vi "Configure Frequency Shift.vi"(0 "niUsrpRio session":T1 {"Daughterboard Clock Rate" format="%#.3pHz"; "FPGA Data Clock Rate" format="%#.3pHz"; "Data Clock Rate" format="%#.3pHz"; "Characterization Data"."Frequencies [Hz]" format="%#_6p"; "EEPROM Characterization Header"."Pointer to Device Data Header" format="%x"; "EEPROM Characterization Header"."Checksum" format="%x"; "Device Data Header"."Pointer to Characterization Data" format="%x"; "Device Data Header"."Checksum" format="%x"; "EEPROM Header"."Pointer to User Header" format="%x"; "EEPROM Header"."Pointer to Factory Header" format="%x"; "EEPROM Header"."Product Code" format="%x"; "EEPROM Header"."Checksum" format="%x"}, 1 "scope":string(combo)="rx", 5 "clock rate":dbl=120000000.0 format="%#.3pHz", 7 "frequency shift":dbl format="%#.3pHz", 11 "error in":errorcluster) -> (4 "niUsrpRio Session (out)":T1={"FPGA Interface"=refnum, "RIO Interface Number"=0, "Data Clock Rate"=0, "FPGA Data Clock Rate"=0, "Global Settings Register Bus"=refnum, "Radio 0 Settings Register Bus"=refnum, "Radio 1 Settings Register Bus"=refnum, "Radio Settings Bus Semaphore"=refnum, "DB Queues"=[], "Characterization Data Valid?"=FALSE, "EEPROM Header"={"Checksum"=0, "Product Code"=0, "Hardware Current Version"=0, "Hardware Oldest Compatible Version"=0, "EEPROM Map Current Version"=0, "EEPROM Map Oldest Compatible Version"=0, "User Password"="", "Pointer to Factory Header"=0, "Pointer to User Header"=0, "Recommended Interval"=0, "Number of Reserved Bytes"=9, "Number of Daughterboards"=0, "Daughterboard IDs"=[], "Daughterboard Serial Numbers"=[]}, "Device Data Header"={"Checksum"=0, "Number of Channels"=0, "Number of Gain Settings"=[], "Pointer to Characterization Data"=[], "Number of Reserved Bytes"=27, "Number of Frequencies"=[]}, "EEPROM Characterization Header"={"Checksum"=0, "Date"=timestamp(0 s since 1904-01-01), "Temperature"=0.0, "Misc. Info"="", "Pointer to Device Data Header"=0, "Number of Reserved Bytes"=28}, "Characterization Data"=[], "FPGA Current Version"=0, "FPGA Oldest Compatible Version"=0, "Fixed Logic Current Version"=0, "Fixed Logic Oldest Compatible Version"=0, "FPGA Radio Settings Bus Current Version"=0, "FPGA Radio Settings Bus Oldest Compatible Version"=0, "FPGA Board Config Current Version"=0, "FPGA Board Config Oldest Compatible Version"=0, "Daughterboard Clock Rate"=0} {"Daughterboard Clock Rate" format="%#.3pHz"; "FPGA Data Clock Rate" format="%#.3pHz"; "Data Clock Rate" format="%#.3pHz"; "Characterization Data"."Frequencies [Hz]" format="%#_6p"; "EEPROM Characterization Header"."Pointer to Device Data Header" format="%x"; "EEPROM Characterization Header"."Checksum" format="%x"; "Device Data Header"."Pointer to Characterization Data" format="%x"; "Device Data Header"."Checksum" format="%x"; "EEPROM Header"."Pointer to User Header" format="%x"; "EEPROM Header"."Pointer to Factory Header" format="%x"; "EEPROM Header"."Product Code" format="%x"; "EEPROM Header"."Checksum" format="%x"}, 8 "coerced frequency shift":dbl format="%#.3pHz", 15 "error out":errorcluster)   [LabVIEW 2015]
doc: "Configures the digital frequency shift amount.\n\n<B>Input Parameters</B>\n\n<B>niUsrpRio Session</B> is the object created by the Open VI and used as the session handle for the USRP RIO design library.\n\n<B>clock rate</B> is the frequency, in hertz, at which the DSP blocks run.\n\n<B>frequency shift</B> is the amount, in hertz, by which to shift the frequency.\n\n<B>error in</B> describes error conditions that occur before this node runs. This input provides standard 'error in' functionality.\n\n<B>Output Parameters</B>\n\n<B>error out</B> contains error information. This output provides standard 'error out' functionality."
uses:
  <instrlib>/niUsrpRio/Config/v1/Host/Public/niUsrpRio Session.ctl
  <instrlib>/_niInstr/Register Bus/v0/Host/Public/Register Bus Session.ctl
  <instrlib>/_niInstr/Register Bus/v0/Host/Private/Session Data.ctl
  <instrlib>/niUsrpRio/Config/v1/Host/Private/DB Queue Reference.ctl
  <instrlib>/niUsrpRio/Config/v1/Host/Private/Daughterboard Data.ctl
  <instrlib>/niUsrpRio/Config/v1/Host/Private/ATR state data.ctl
  <instrlib>/niUsrpRio/Config/v1/Host/Private/Antenna Configuration.ctl
  <instrlib>/niUsrpRio/Config/v1/Host/Private/CPLD Power Mode.ctl
  <instrlib>/niUsrpRio/Config/v1/Host/Public/EEPROM Header.ctl
  <instrlib>/niUsrpRio/Config/v1/Host/Public/EEPROM Device Data Header.ctl
  <instrlib>/niUsrpRio/Config/v1/Host/Public/EEPROM Characterization Header.ctl
  <instrlib>/niUsrpRio/Config/v1/Host/Public/Characterization Data.ctl
  <instrlib>/niUsrpRio/Config/v1/Host/Public/IQ Imbalance.ctl
  Streaming Xvcr FPGA Ref.ctl
  FPGA/SubVIs/DDC Parameters.ctl
  <instrlib>/_niInstr/DSP/v1/Shared/Public/IQ Impairments.ctl
  <vilib>/rvi/errors/niLvFpgaAdjustHostInterfaceError.vi
  <vilib>/Utility/error.llb/Error Cluster From Error Code.vi
  <vilib>/rvi/interface/nirviReadWriteControl/nirviReadWriteControl.xnode
  NiFpgaLv.dll
  <vilib>/rvi/interface/Simulation/niFpgaSimulationCallBeginRW.vi
  <instrlib>/niUsrpRio/Config/v1/Host/niUsrpRio Config v1 Host.lvlib
  <instrlib>/_niInstr/DSP/v1/Shared/niInstr DSP v1 Shared.lvlib
  <instrlib>/_niInstr/Register Bus/v0/Host/niInstr Register Bus v0 Host.lvlib
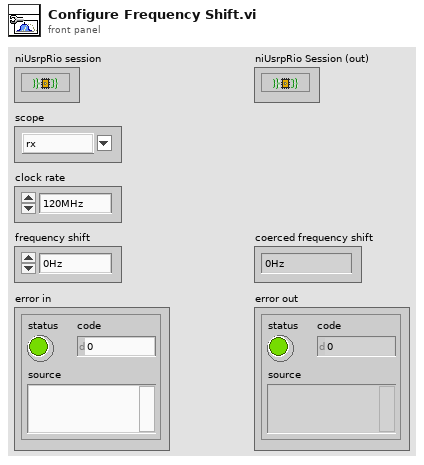
[diagram p1: front panel]
types:
  T1 = typedef "niUsrpRio Config v1 Host.lvlib/niUsrpRio Session.ctl" = cluster{"FPGA Interface":refnum<k20>, "RIO Interface Number":u32, "Data Clock Rate":u32, "FPGA Data Clock Rate":u32, "Global Settings Register Bus":T2, "Radio 0 Settings Register Bus":T2, "Radio 1 Settings Register Bus":T2, "Radio Settings Bus Semaphore":T3, "DB Queues":T4[], "Characterization Data Valid?":bool, "EEPROM Header":T5, "Device Data Header":T6, "EEPROM Characterization Header":T7, "Characterization Data":T8[], "FPGA Current Version":u32, "FPGA Oldest Compatible Version":u32, "Fixed Logic Current Version":u32, "Fixed Logic Oldest Compatible Version":u32, "FPGA Radio Settings Bus Current Version":u32, "FPGA Radio Settings Bus Oldest Compatible Version":u32, "FPGA Board Config Current Version":u32, "FPGA Board Config Oldest Compatible Version":u32, "Daughterboard Clock Rate":u32}
  T2 = typedef "niInstr Register Bus v0 Host.lvlib/Register Bus Session.ctl" = refnum<queue>
  T3 = typedef "Semaphore RefNum" = refnum<k1>
  T4 = typedef "niUsrpRio Config v1 Host.lvlib/DB Queue Reference.ctl" = refnum<queue>
  T5 = typedef "niUsrpRio Config v1 Host.lvlib/EEPROM Header.ctl" = cluster{"Checksum":u32, "Product Code":u16, "Hardware Current Version":u16, "Hardware Oldest Compatible Version":u16, "EEPROM Map Current Version":u16, "EEPROM Map Oldest Compatible Version":u16, "User Password":string, "Pointer to Factory Header":u32, "Pointer to User Header":u32, "Recommended Interval":u16, "Number of Reserved Bytes":i32, "Number of Daughterboards":u8, "Daughterboard IDs":u16[], "Daughterboard Serial Numbers":string[]}
  T6 = typedef "niUsrpRio Config v1 Host.lvlib/EEPROM Device Data Header.ctl" = cluster{"Checksum":u32, "Number of Channels":u8, "Number of Gain Settings":u16[], "Pointer to Characterization Data":u32[], "Number of Reserved Bytes":i32, "Number of Frequencies":u16[]}
  T7 = typedef "niUsrpRio Config v1 Host.lvlib/EEPROM Characterization Header.ctl" = cluster{"Checksum":u32, "Date":timestamp, "Temperature":sgl, "Misc. Info":string, "Pointer to Device Data Header":u32, "Number of Reserved Bytes":i32}
  T8 = typedef "niUsrpRio Config v1 Host.lvlib/Characterization Data.ctl" = cluster{"Gains[dB]":dbl[], "Frequencies [Hz]":dbl[], "IQ Imbalance Table":T9[], "Measured Gains[dB]":dbl[][]}
  T9 = typedef "niUsrpRio Config v1 Host.lvlib/IQ Imbalance.ctl" = cluster{"Gain Imbalance [linear]":dbl, "Phase Imbalance [radians]":dbl, "Offset":cdb}
  T10 = typedef "DDC Parameters.ctl" = cluster{"output sample rate":fxp<+,48,1>, "delay":fxp<+/-,16,0>, "frequency shift":fxp<+/-,48,0>, "impairments":T11, "phase":fxp<+/-,21,0>}
  T11 = typedef "niInstr DSP v1 Shared.lvlib/IQ Impairments.ctl" = cluster{"inline gain I":fxp<+/-,18,1>, "inline gain Q":fxp<+/-,18,1>, "cross gain I":fxp<+/-,18,1>, "cross gain Q":fxp<+/-,18,1>, "pre-gain offset I":fxp<+/-,18,1>, "pre-gain offset Q":fxp<+/-,18,1>, "post-gain offset I":fxp<+/-,18,1>, "post-gain offset Q":fxp<+/-,18,1>}
  T12 = typedef "Streaming Xvcr FPGA Ref.ctl" = refnum<k20>
  T13 = typedef "niUsrpRio Config v1 Host.lvlib/Device Subfunction.ctl" = enum16{"rx", "tx", "all"}
  T14 = typedef "niUsrpRio Config v1 Host.lvlib/RF Channel.ctl" = enum16{"0", "1", "All"}
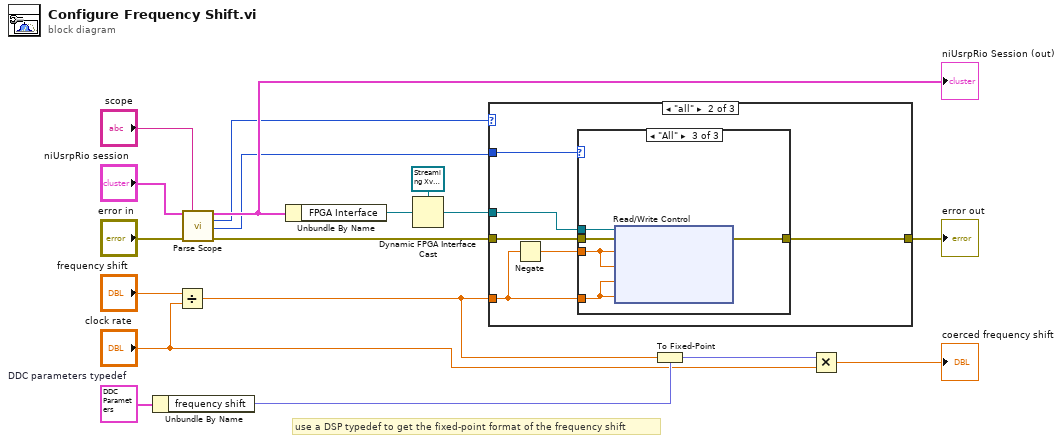
[diagram p0: block diagram]
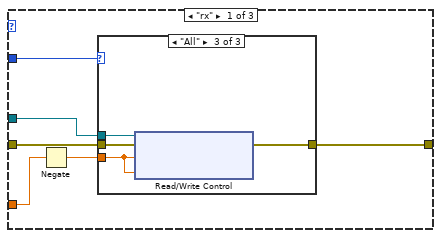
[diagram p2: hidden frame]
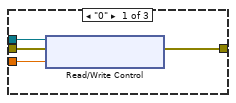
[diagram p3: hidden frame]
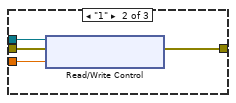
[diagram p4: hidden frame]
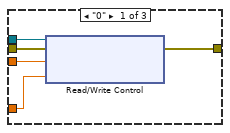
[diagram p5: hidden frame]
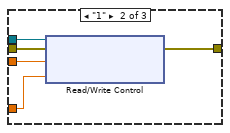
[diagram p6: hidden frame]
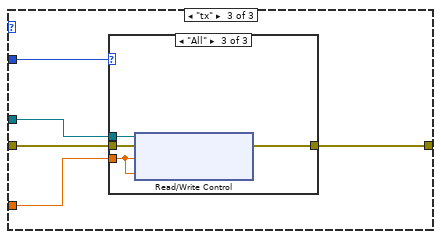
[diagram p7: hidden frame]
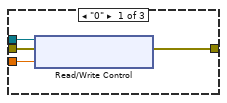
[diagram p8: hidden frame]
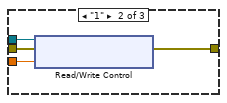
[diagram p9: hidden frame]
diagram:
  w6 = T10 {"output sample rate"=1.0, "delay"=0.0, "frequency shift"=0.0, "impairments"={"inline gain I"=0.9999923706054688, "inline gain Q"=0.9999923706054688, "cross gain I"=0.0, "cross gain Q"=0.0, "pre-gain offset I"=0.0, "pre-gain offset Q"=0.0, "post-gain offset I"=0.0, "post-gain offset Q"=0.0}, "phase"=0.0}  # DDC parameters typedef
  # "use a DSP typedef to get the fixed-point format of the frequency shift"
  n1 = Unbundle By Name(w6) -> ("frequency shift"=w2:fxp<+/-,48,0>)
  n2 = Divide(x="frequency shift", y="clock rate") -> (x/y=w4:dbl)
  n3 = call <instrlib>:"Parse Scope.vi"("niUsrpRio Session"="niUsrpRio session", "scope"="scope", "error in"="error in") -> ("niUsrpRio Session (out)"=w18:T1, "Device Subfunction"=w15:T13, "Device Subfunction Channel"=w16:T14, "error out"=w17:errorcluster)  [unwired: 4 in, 5 out]
  "niUsrpRio Session (out)" <- w18
  n4 = Unbundle By Name(w18) -> ("FPGA Interface"=w8:refnum<k20>)
  n5 = Dynamic FPGA Interface Cast(Session In=T12 refnum ("FPGA VI Reference Out"), Type=w8) -> (Session Out=w7:T12)
  n6 = case shown="\"all\"" w15 {
    tunnel: w4 -> [w19 w37 w58]
    tunnel: w7 -> [w20 w38 w62]
    tunnel: [w24 w42 w61] -> w10
    tunnel: w17 -> [w23 w41 w60]
    tunnel: w16 -> [w21 w39 w59]
    frame "rx" {
      n7 = Negate(x=w19) -> (-x=w22:dbl)
      n8 = case shown="\"All\"" w21 {
        tunnel: w20 -> [w28 w32 w36]
        tunnel: [w27 w31 w35] -> w24
        tunnel: w23 -> [w26 w30 w34]
        tunnel: w22 -> [w25 w29 w33]
        frame "0" {
          n9 = xnode "Read/Write Control"("FPGA VI Reference In"=w28, "error in"=w26, "rx 0.frequency shift"=w25) -> ("error out"=w27:errorcluster)  [unwired: 1 out]
        }
        frame "1" {
          n10 = xnode "Read/Write Control"("FPGA VI Reference In"=w32, "error in"=w30, "rx 1.frequency shift"=w29) -> ("error out"=w31:errorcluster)  [unwired: 1 out]
        }
        frame "All" {
          n11 = xnode "Read/Write Control"("FPGA VI Reference In"=w36, "error in"=w34, "rx 0.frequency shift"=w33, "rx 1.frequency shift"=w33) -> ("error out"=w35:errorcluster)  [unwired: 1 out]
        }
      }
    }
    frame "all" {
      n12 = Negate(x=w37) -> (-x=w40:dbl)
      n13 = case shown="\"All\"" w39 {
        tunnel: w38 -> [w47 w52 w57]
        tunnel: [w46 w51 w56] -> w42
        tunnel: w41 -> [w45 w50 w55]
        tunnel: w40 -> [w44 w49 w54]
        tunnel: w37 -> [w43 w48 w53]
        frame "0" {
          n14 = xnode "Read/Write Control"("FPGA VI Reference In"=w47, "error in"=w45, "rx 0.frequency shift"=w44, "tx 0.frequency shift"=w43) -> ("error out"=w46:errorcluster)  [unwired: 1 out]
        }
        frame "1" {
          n15 = xnode "Read/Write Control"("FPGA VI Reference In"=w52, "error in"=w50, "rx 1.frequency shift"=w49, "tx 1.frequency shift"=w48) -> ("error out"=w51:errorcluster)  [unwired: 1 out]
        }
        frame "All" {
          n16 = xnode "Read/Write Control"("FPGA VI Reference In"=w57, "error in"=w55, "rx 0.frequency shift"=w54, "rx 1.frequency shift"=w54, "tx 0.frequency shift"=w53, "tx 1.frequency shift"=w53) -> ("error out"=w56:errorcluster)  [unwired: 1 out]
        }
      }
    }
    frame "tx" {
      n17 = case shown="\"All\"" w59 {
        tunnel: w58 -> [w66 w70 w71]
        tunnel: w62 -> [w65 w69 w74]
        tunnel: [w64 w68 w73] -> w61
        tunnel: w60 -> [w63 w67 w72]
        frame "0" {
          n18 = xnode "Read/Write Control"("FPGA VI Reference In"=w65, "error in"=w63, "tx 0.frequency shift"=w66) -> ("error out"=w64:errorcluster)  [unwired: 1 out]
        }
        frame "1" {
          n19 = xnode "Read/Write Control"("FPGA VI Reference In"=w69, "error in"=w67, "tx 1.frequency shift"=w70) -> ("error out"=w68:errorcluster)  [unwired: 1 out]
        }
        frame "All" {
          n20 = xnode "Read/Write Control"("FPGA VI Reference In"=w74, "error in"=w72, "tx 0.frequency shift"=w71, "tx 1.frequency shift"=w71) -> ("error out"=w73:errorcluster)  [unwired: 1 out]
        }
      }
    }
  }
  "error out" <- w10
  n21 = To Fixed-Point(fixed-point type=w2, number=w4) -> (fixed-point=w5:fxp<+/-,48,0>)
  n22 = Multiply(x=w5, y="clock rate") -> (x*y=→"coerced frequency shift":dbl)
